vi "seletor_adq.vi"(3 "Valvulas":T1, 5 "Matriz entrada":dbl[][](array[numeric])) -> (1 "matriz saída":dbl[][](array[numeric]))   [LabVIEW 2019]
panel:
  out "appended array":dbl[][](array[numeric])
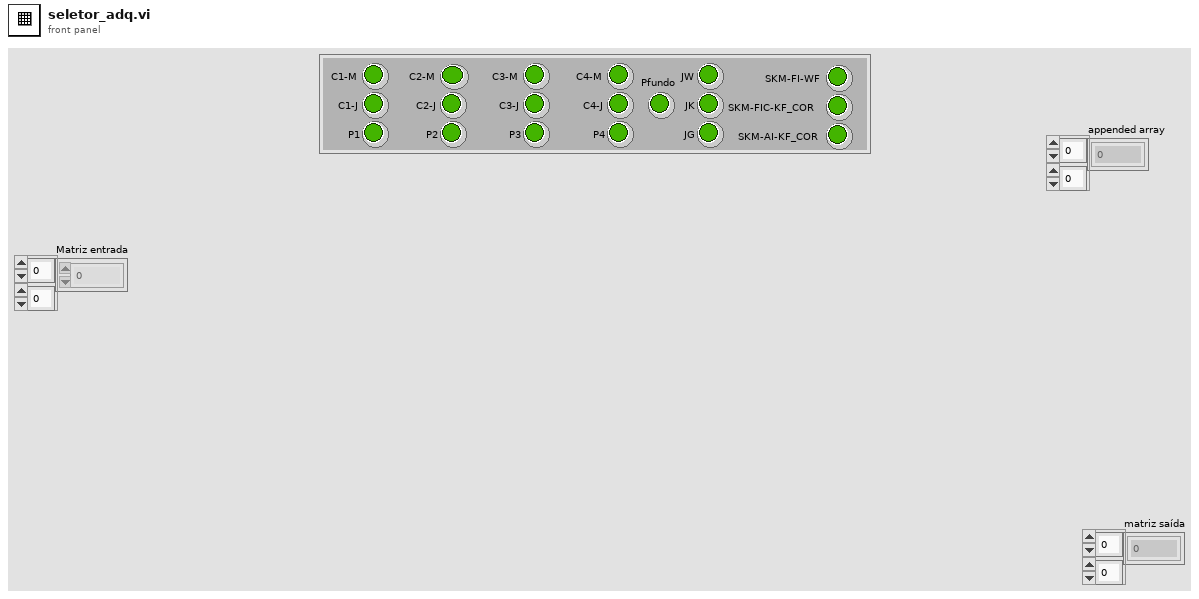
[diagram p1: front panel]
types:
  T1 = cluster{"C1-M":bool, "C1-J":bool, "P1":bool, "C2-M":bool, "C2-J":bool, "P2":bool, "C3-M":bool, "C3-J":bool, "P3":bool, "C4-M":bool, "C4-J":bool, "P4":bool, "Pfundo":bool, "JW":bool, "JK":bool, "JG":bool, "SKM-FI-WF":bool, "SKM-FIC-KF_COR":bool, "SKM-AI-KF_COR":bool}
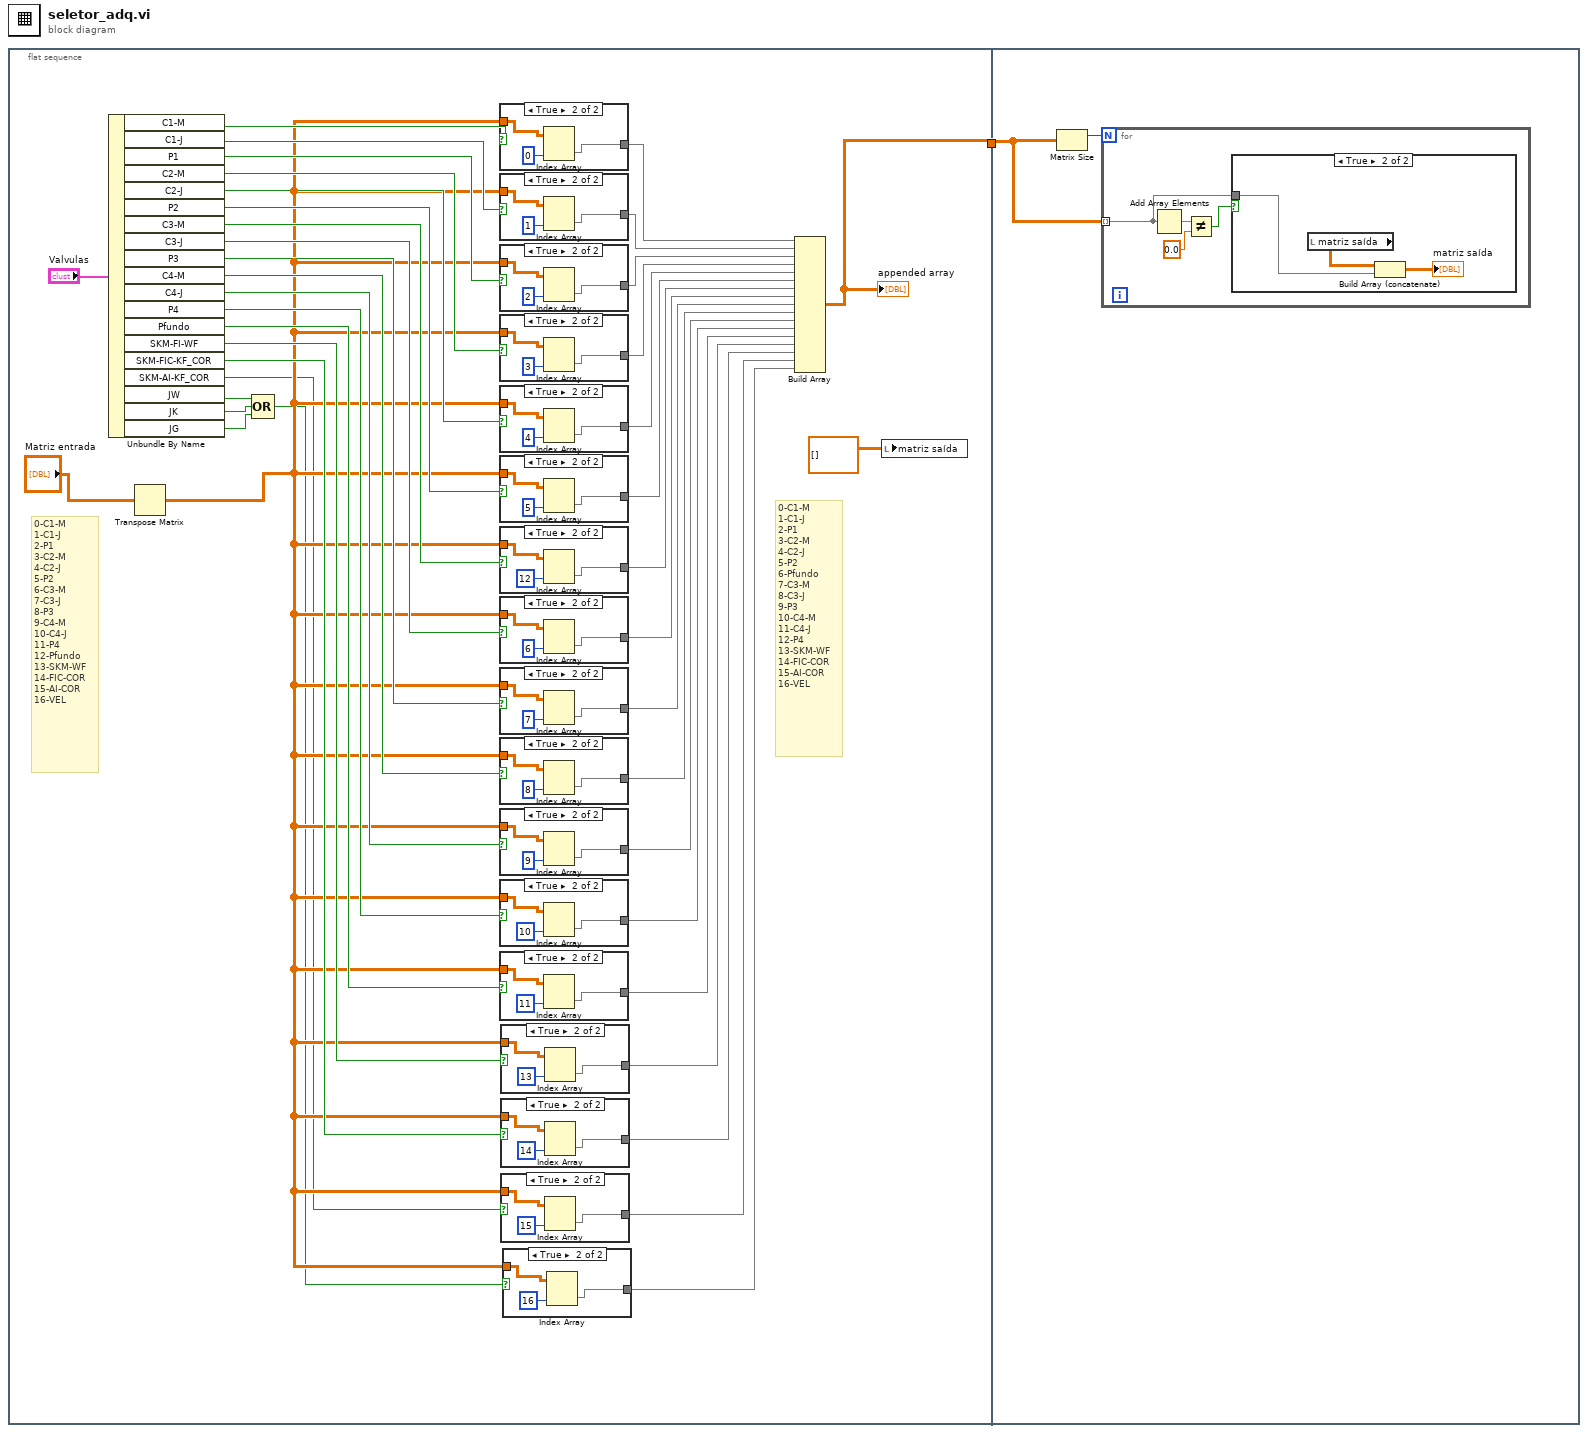
[diagram p0: block diagram]
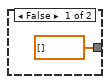
[diagram p2: hidden frame]
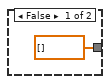
[diagram p3: hidden frame]
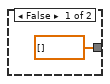
[diagram p4: hidden frame]
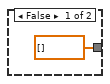
[diagram p5: hidden frame]
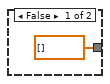
[diagram p6: hidden frame]
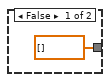
[diagram p7: hidden frame]
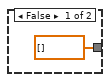
[diagram p8: hidden frame]
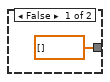
[diagram p9: hidden frame]
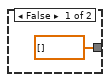
[diagram p10: hidden frame]
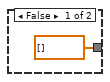
[diagram p11: hidden frame]
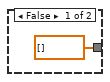
[diagram p12: hidden frame]
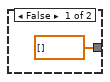
[diagram p13: hidden frame]
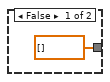
[diagram p14: hidden frame]
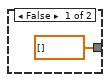
[diagram p15: hidden frame]
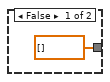
[diagram p16: hidden frame]
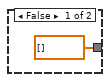
[diagram p17: hidden frame]
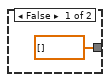
[diagram p18: hidden frame]
diagram:
  n1 = flat-sequence {
    tunnel: [w17] -> w1
    tunnel: w1 -> [w112]
    frame #0 {
      # "0-C1-M\n1-C1-J\n2-P1\n3-C2-M\n4-C2-J\n5-P2\n6-Pfundo\n7-C3-M\n8-C3-J\n9-P3\n10-C4-M\n11-C4-J\n12-P4\n13-SKM-WF\n14-FIC-COR\n15-AI-COR\n16-VEL"
      # "0-C1-M\n1-C1-J\n2-P1\n3-C2-M\n4-C2-J\n5-P2\n6-C3-M\n7-C3-J\n8-P3\n9-C4-M\n10-C4-J\n11-P4\n12-Pfundo\n13-SKM-WF\n14-FIC-COR\n15-AI-COR\n16-VEL"
      n2 = Unbundle By Name("Valvulas") -> ("C1-M"=w30:bool, "C1-J"=w29:bool, "P1"=w28:bool, "C2-M"=w27:bool, "C2-J"=w26:bool, "P2"=w25:bool, "C3-M"=w24:bool, "C3-J"=w23:bool, "P3"=w22:bool, "C4-M"=w21:bool, "C4-J"=w20:bool, "P4"=w19:bool, "Pfundo"=w18:bool, "SKM-FI-WF"=w14:bool, "SKM-FIC-KF_COR"=w13:bool, "SKM-AI-KF_COR"=w11:bool, "JW"=w10:bool, "JK"=w9:bool, "JG"=w8:bool)
      n3 = Transpose Matrix(1:"Matriz entrada") -> (0:w12:dbl[][])
      n4 = Compound Arithmetic op=OR(w10, w9, w8) -> (w7:bool)
      n5 = case shown="True" w30 {
        tunnel: w12 -> [_ w111]
        tunnel: [dbl[] [] ("Matriz") w109] -> w43
        frame False {
        }
        frame True {
          n6 = Index Array(array=w111, index (col)=0 ("disabled index (col)")) -> (element=w109:dbl[])  [unwired: 1 in]
        }
      }
      n7 = case shown="True" w29 {
        tunnel: w12 -> [_ w107]
        tunnel: [dbl[] [] ("Matriz") w105] -> w42
        frame False {
        }
        frame True {
          n8 = Index Array(array=w107, index (col)=1 ("disabled index (col)")) -> (element=w105:dbl[])  [unwired: 1 in]
        }
      }
      n9 = case shown="True" w28 {
        tunnel: w12 -> [_ w103]
        tunnel: [dbl[] [] ("Matriz") w101] -> w41
        frame False {
        }
        frame True {
          n10 = Index Array(array=w103, index (col)=2 ("disabled index (col)")) -> (element=w101:dbl[])  [unwired: 1 in]
        }
      }
      n11 = case shown="True" w27 {
        tunnel: w12 -> [_ w99]
        tunnel: [dbl[] [] ("Matriz") w97] -> w40
        frame False {
        }
        frame True {
          n12 = Index Array(array=w99, index (col)=3 ("disabled index (col)")) -> (element=w97:dbl[])  [unwired: 1 in]
        }
      }
      n13 = case shown="True" w26 {
        tunnel: w12 -> [_ w95]
        tunnel: [dbl[] [] ("Matriz") w93] -> w39
        frame False {
        }
        frame True {
          n14 = Index Array(array=w95, index (col)=4 ("disabled index (col)")) -> (element=w93:dbl[])  [unwired: 1 in]
        }
      }
      n15 = case shown="True" w25 {
        tunnel: w12 -> [_ w91]
        tunnel: [dbl[] [] ("Matriz") w89] -> w38
        frame False {
        }
        frame True {
          n16 = Index Array(array=w91, index (col)=5 ("disabled index (col)")) -> (element=w89:dbl[])  [unwired: 1 in]
        }
      }
      n17 = case shown="True" w24 {
        tunnel: w12 -> [_ w87]
        tunnel: [dbl[] [] ("Matriz") w85] -> w37
        frame False {
        }
        frame True {
          n18 = Index Array(array=w87, index (col)=12 ("disabled index (col)")) -> (element=w85:dbl[])  [unwired: 1 in]
        }
      }
      n19 = case shown="True" w23 {
        tunnel: w12 -> [_ w83]
        tunnel: [dbl[] [] ("Matriz") w81] -> w36
        frame False {
        }
        frame True {
          n20 = Index Array(array=w83, index (col)=6 ("disabled index (col)")) -> (element=w81:dbl[])  [unwired: 1 in]
        }
      }
      n21 = case shown="True" w22 {
        tunnel: w12 -> [_ w79]
        tunnel: [dbl[] [] ("Matriz") w77] -> w35
        frame False {
        }
        frame True {
          n22 = Index Array(array=w79, index (col)=7 ("disabled index (col)")) -> (element=w77:dbl[])  [unwired: 1 in]
        }
      }
      n23 = case shown="True" w21 {
        tunnel: w12 -> [_ w75]
        tunnel: [dbl[] [] ("Matriz") w73] -> w34
        frame False {
        }
        frame True {
          n24 = Index Array(array=w75, index (col)=8 ("disabled index (col)")) -> (element=w73:dbl[])  [unwired: 1 in]
        }
      }
      n25 = case shown="True" w20 {
        tunnel: w12 -> [_ w71]
        tunnel: [dbl[] [] ("Matriz") w69] -> w33
        frame False {
        }
        frame True {
          n26 = Index Array(array=w71, index (col)=9 ("disabled index (col)")) -> (element=w69:dbl[])  [unwired: 1 in]
        }
      }
      n27 = case shown="True" w19 {
        tunnel: w12 -> [_ w67]
        tunnel: [dbl[] [] ("Matriz") w65] -> w32
        frame False {
        }
        frame True {
          n28 = Index Array(array=w67, index (col)=10 ("disabled index (col)")) -> (element=w65:dbl[])  [unwired: 1 in]
        }
      }
      n29 = case shown="True" w18 {
        tunnel: w12 -> [_ w63]
        tunnel: [dbl[] [] ("Matriz") w61] -> w31
        frame False {
        }
        frame True {
          n30 = Index Array(array=w63, index (col)=11 ("disabled index (col)")) -> (element=w61:dbl[])  [unwired: 1 in]
        }
      }
      n31 = case shown="True" w14 {
        tunnel: w12 -> [_ w59]
        tunnel: [dbl[] [] ("Matriz") w57] -> w6
        frame False {
        }
        frame True {
          n32 = Index Array(array=w59, index (col)=13 ("disabled index (col)")) -> (element=w57:dbl[])  [unwired: 1 in]
        }
      }
      n33 = case shown="True" w13 {
        tunnel: w12 -> [_ w55]
        tunnel: [dbl[] [] ("Matriz") w53] -> w5
        frame False {
        }
        frame True {
          n34 = Index Array(array=w55, index (col)=14 ("disabled index (col)")) -> (element=w53:dbl[])  [unwired: 1 in]
        }
      }
      n35 = case shown="True" w11 {
        tunnel: w12 -> [_ w51]
        tunnel: [dbl[] [] ("Matriz") w49] -> w4
        frame False {
        }
        frame True {
          n36 = Index Array(array=w51, index (col)=15 ("disabled index (col)")) -> (element=w49:dbl[])  [unwired: 1 in]
        }
      }
      n37 = case shown="True" w7 {
        tunnel: w12 -> [_ w47]
        tunnel: [dbl[] [] ("Matriz") w45] -> w3
        frame False {
        }
        frame True {
          n38 = Index Array(array=w47, index (col)=16 ("disabled index (col)")) -> (element=w45:dbl[])  [unwired: 1 in]
        }
      }
      n39 = Build Array(w43, w42, w41, w40, w39, w38, w37, w36, w35, w34, w33, w32, w31, w6, w5, w4, w3) -> (w17:dbl[][])
      "appended array" <- w17
      n40 = local write "matriz saída"(dbl[][] [] ("appended array 2")) -> ()
    }
    frame #1 {
      n41 = Matrix Size(0:w112) -> (1:w113:i32)  [unwired: 1 out]
      n42 = for {
        N: w113 -> [_]
        tunnel: w112 -> [w114] mode=indexing
        n43 = Add Array Elements(numeric array=w114) -> (sum=w117:dbl)
        n44 = Not Equal?(x=w117, y=0.0) -> (x != y?=w115:bool)
        n45 = case shown="True" w115 {
          tunnel: w114 -> [_ w120]
          frame False {
          }
          frame True {
            n46 = local read "matriz saída"() -> (w118:dbl[][])
            n47 = Build Array (concatenate)(w118, w120) -> (→"matriz saída":dbl[][])
          }
        }
      }
    }
  }
